vi "PicoScope2000aSetDataBuffers.vi"(5 "enabled array":i16[](array[numeric]), 7 "Buffer and Transfer Settings":T3={"startIndex"=0, "Samples"=1000, "Down Sample Ratio"=1, "Down-Sample Mode"=1} {"Down-Sample Mode" items=["RAW none"=2147483648, "None"=0, "Aggregate"=1, "Decimate"=2, "Average"=4]; "Down Sample Ratio" step=1; "Samples" format="%_6p"}, 8 "error in (no error)":errorcluster, 9 "Device Info":T1={"Driver Version"="2.1.104.3324", "USB Version"="2.0", "Hardware"="1", "Variant"="2206A", "Batch and Serial"="CV676/049", "Cal Date"="19Sep17", "Kernel Version"="1.0", "Digital HW Version"="1", "Analogue HW Version"="1", "Firmware 1"="1.3.3.0", "Firmware 2"="0.5.47.0", "MSO"=FALSE, "Number of Channels"=2}, 10 "Data Pointers In":T2, 11 "handle in":i16) -> (0 "error out":errorcluster, 3 "handle out":i16)   [LabVIEW 2010]
doc: "Calls SetDataBuffers, and assigns Pico buffers"
uses:
  ps2000a.dll
  shared/PicoBuffers.ctl
  shared/Buffer and Transfer Settings.ctl
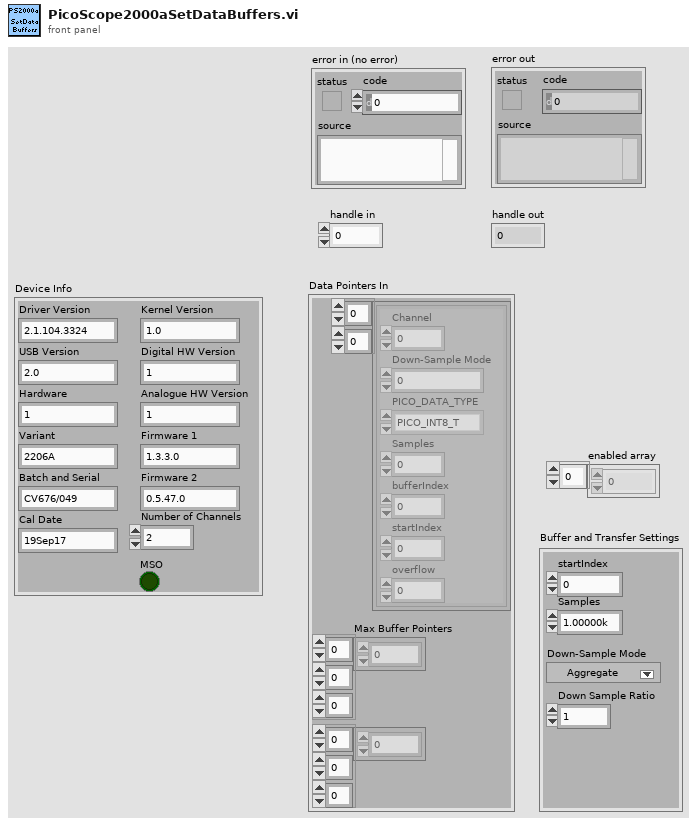
[diagram p1: front panel]
types:
  T1 = cluster{"Driver Version":string, "USB Version":string, "Hardware":string, "Variant":string, "Batch and Serial":string, "Cal Date":string, "Kernel Version":string, "Digital HW Version":string, "Analogue HW Version":string, "Firmware 1":string, "Firmware 2":string, "MSO":bool, "Number of Channels":i16}
  T2 = typedef "PicoBuffers.ctl" = cluster{"Max Buffer Pointers":u64[][][], "Min Buffer Pointers":u64[][][], "StreamingDataInfo":cluster{"Channel":u32, "Down-Sample Mode":u32, "PICO_DATA_TYPE":enum32{"PICO_INT8_T", "PICO_INT16_T", "PICO_INT32_T", "PICO_UINT32_T", "PICO_INT64_T", ""}, "Samples":i32, "bufferIndex":u64, "startIndex":i32, "overflow":i16}[][]}
  T3 = typedef "Buffer and Transfer Settings.ctl" = cluster{"startIndex":u64, "Samples":u64, "Down Sample Ratio":u64, "Down-Sample Mode":u32}
  T4 = cluster{"status":bool, "code":u32, "source":string}
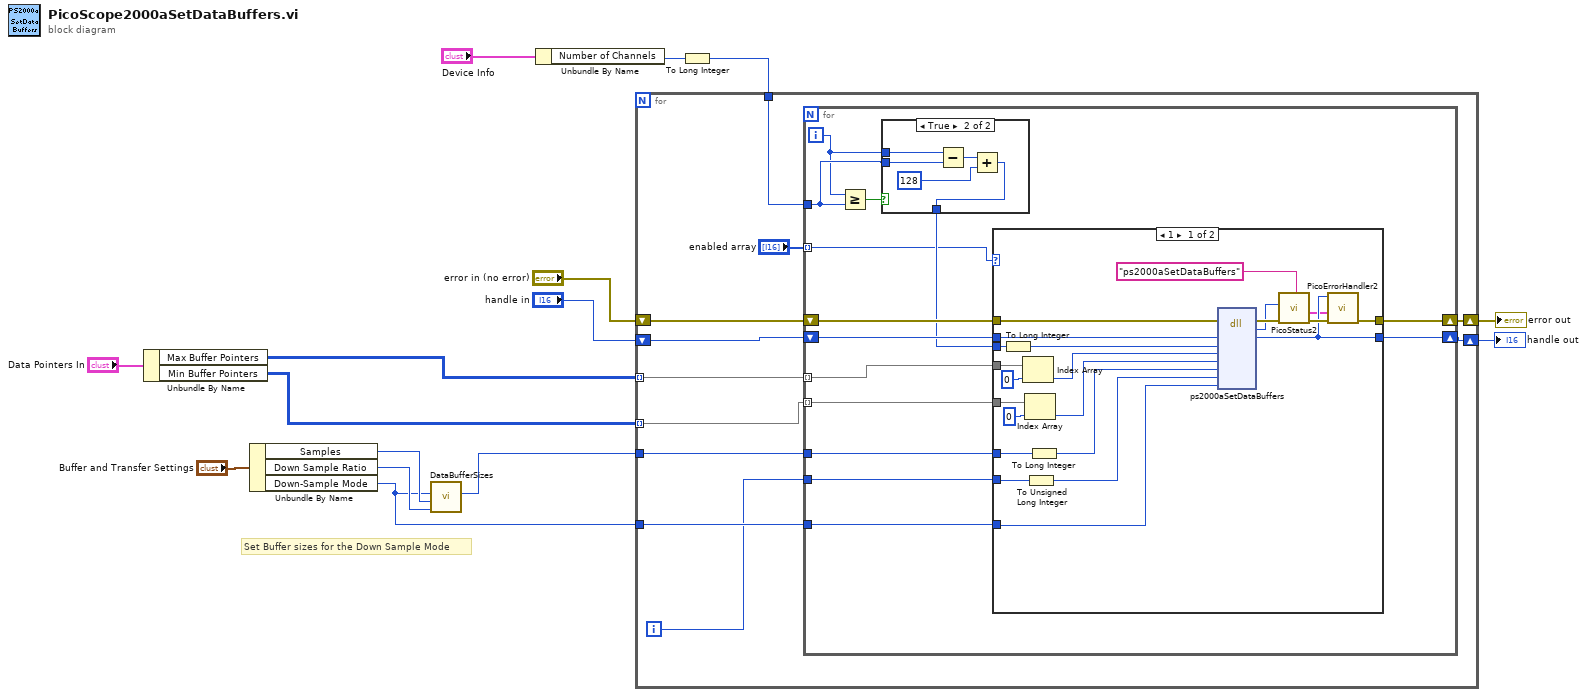
[diagram p0: block diagram]
diagram:
  # "Set Buffer sizes for the Down Sample Mode"
  n1 = Unbundle By Name("Data Pointers In") -> ("Max Buffer Pointers"=w5:u64[][][], "Min Buffer Pointers"=w4:u64[][][])
  n2 = Unbundle By Name("Buffer and Transfer Settings") -> ("Samples"=w7:u64, "Down Sample Ratio"=w8:u64, "Down-Sample Mode"=w6:u32)
  n3 = call "DataBufferSizes.vi"("Down Sample Ratio"=w8, "Number of Samples"=w7, "Down-Sample Mode"=w6) -> ("Max Buffer Size"=w9:i32)  [unwired: 7 in, 1 out]
  n4 = Unbundle By Name("Device Info") -> ("Number of Channels"=w3:i16)
  n5 = To Long Integer(number=w3) -> (32bit integer=w1:i32)
  n6 = for {
    tunnel: w9 -> [w22]
    tunnel: w6 -> [w21]
    tunnel: w5 -> [w20] mode=indexing
    tunnel: w4 -> [w19] mode=indexing
    shift-right: [w26] -> w14
    shift-left: "error in (no error)" -> [w24]
    shift-right: [w25] -> w13
    shift-left: "handle in" -> [w23]
    tunnel: w1 -> [w16]
    i -> [w17]
    n7 = for {
      tunnel: w21 -> [w40]
      tunnel: w22 -> [w37]
      tunnel: "enabled array" -> [w27] mode=indexing
      tunnel: w20 -> [w36] mode=indexing
      shift-right: [w35] -> w26
      shift-left: w24 -> [w39]
      tunnel: w19 -> [w34] mode=indexing
      shift-right: [w33] -> w25
      shift-left: w23 -> [w38]
      tunnel: w17 -> [w32]
      tunnel: w16 -> [w30]
      i -> [w29]
      n8 = Greater Or Equal?(x=w29, y=w30) -> (x >= y?=w31:bool)
      n9 = case shown="True" w31 {
        tunnel: [w41 w45] -> w28
        tunnel: w30 -> [_ w44]
        tunnel: w29 -> [w41 w43]
        frame False {
        }
        frame True {
          n10 = Subtract(x=w43, y=w44) -> (x-y=w42:i32)
          n11 = Add(x=w42, y=128) -> (x+y=w45:i32)
        }
      }
      n12 = case shown="1" w27 {
        tunnel: w28 -> [w58 _]
        tunnel: w39 -> [w68 w70]
        tunnel: w38 -> [w65 w69]
        tunnel: w40 -> [w50 _]
        tunnel: [w62 w70] -> w35
        tunnel: [w61 w69] -> w33
        tunnel: w37 -> [w60 _]
        tunnel: w36 -> [w54 _]
        tunnel: w34 -> [w51 _]
        tunnel: w32 -> [w49 _]
        frame 1 {
          n13 = To Long Integer(number=w58) -> (32bit integer=w57:i32)
          n14 = Index Array(array=w54, index=0) -> (element=w55:u64)
          n15 = Index Array(array=w51, index=0) -> (element=w52:u64)
          n16 = To Unsigned Long Integer(number=w49) -> (unsigned 32bit integer=w48:u32)
          n17 = To Long Integer(number=w60) -> (32bit integer=w59:i32)
          n18 = dll-call lib="ps2000a.dll" fn="ps2000aSetDataBuffers" ("ps3000.dll:_ps3000_open_unit@0")(error in=w68, "handle"=w65, "channel"=w57, "bufferMax"=w55, "bufferMin"=w52, "bufferLth"=w59, "segmentIndex"=w48, "downSampleRatioMode"=w50) -> (error out=w67:errorcluster, "PICO_STATUS"=w66:u32, "handle"=w61:i16)  [unwired: 8 in, 1 out]
          n19 = call "PicoStatus2.vi"("PICO source"="ps2000aSetDataBuffers" ("source"), "Error in"=w67, "PICO STATUS"=w66) -> ("error out"=w63:errorcluster, "PICO_STATUS out"=w47:T4)  [unwired: 5 in]
          n20 = call "PicoErrorHandler2.vi"("error in (no error)"=w63, "PICO_STATUS in"=w47, "handle In"=w61) -> ("error out"=w62:errorcluster)  [unwired: 8 in]
        }
        frame 0, Default {
        }
      }
    }
  }
  "error out" <- w14
  "handle out" <- w13
